vi "Manip3.vi"() -> ()   [LabVIEW 2021]
panel:
  in  "Echelle\n\n°C\n\nK":bool=TRUE
  out "Thermometer":dbl(slide) scale=0.0..100.0
  out "x":dbl
  out "?":dbl(slide) scale=0.0..200.0
  out "Temperature":dbl
  in  "Echelle\n\n °F\n\n °C":bool
  in  "Tension":dbl
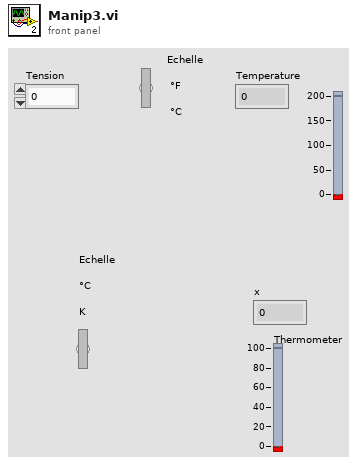
[diagram p1: front panel]
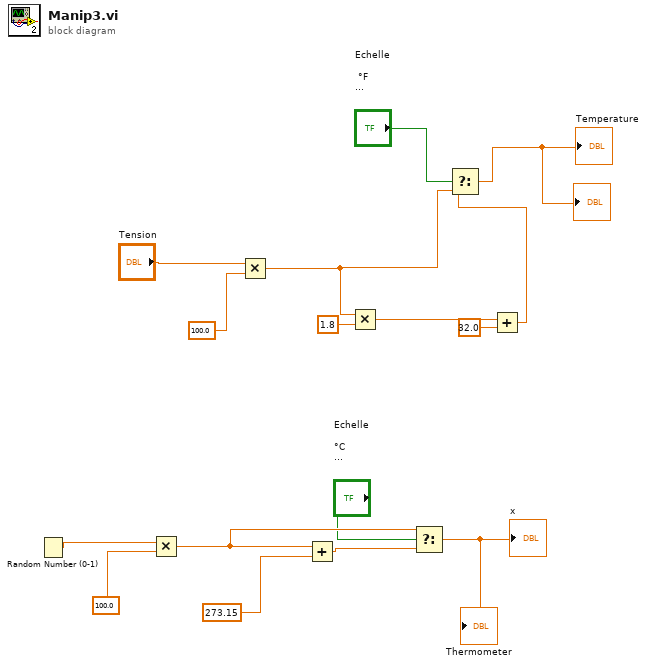
[diagram p0: block diagram]
diagram:
  n1 = Random Number (0-1)() -> (number: 0 to 1=w7:dbl)
  n2 = Multiply(x=w7, y=100.0 ("x")) -> (x*y=w3:dbl)
  n3 = Multiply(x="Tension", y=100.0) -> (x*y=w11:dbl)
  n4 = Add(x=w3, y=273.15) -> (x+y=w4:dbl)
  n5 = Multiply(x=w11, y=1.8) -> (x*y=w15:dbl)
  n6 = Select(t=w3, s="Echelle\n\n°C\n\nK", f=w4) -> (s? t:f=→"x" →"Thermometer":dbl)
  n7 = Add(x=w15, y=32.0) -> (x+y=w12:dbl)
  n8 = Select(t=w12, s="Echelle\n\n °F\n\n °C", f=w11) -> (s? t:f=→"Temperature" →"?":dbl)
